vi "Reconnect.vi"(8 "error in (no error)":errorcluster, 11 "navX - I2C in":refnum<class "navX - I2C.lvclass">) -> (0 "error out":errorcluster, 3 "navX - I2C out":refnum<class "navX - I2C.lvclass">)   [LabVIEW 2015, in "navX Library v3.lvlib" / "navX - I2C.lvclass"]
uses:
  navX - I2C.lvclass
  navX - I2C.lvclass/navX - I2C.ctl
  navX - SPI_I2C ProcessingLoop/navX - SPI_I2C ProcessingLoop.lvclass
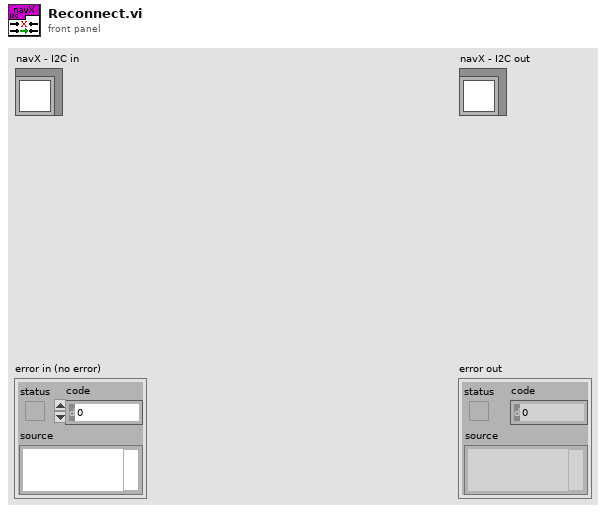
[diagram p1: front panel]
types:
  T1 = typedef "i2c_bus.ctl" = enum16{"I2C On-Board", "I2C MXP", "Invalid"}
  T2 = typedef "WPI_I2CDevRef.ctl" = cluster{"DevStatus":errorcluster, "Device Address":u8, "Handle":i32, "I2C Bus":T1}
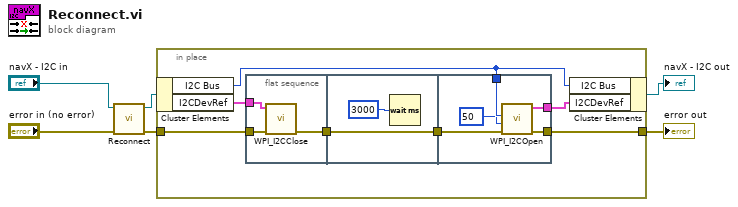
[diagram p0: block diagram]
diagram:
  n1 = call-parent "Reconnect.vi"("error in (no error)"="error in (no error)", "navX - Interface in"="navX - I2C in") -> ("error out"=w3:errorcluster, "navX - Interface out"=w4:refnum<class "navX - I2C.lvclass">)  [unwired: 8 in]
  n2 = in-place {
    in-place-border: [w13] -> w1
    in-place-border: w3 -> [w12]
    n3 = in-place-cluster #1(w4) -> ("I2C Bus"=w9:T1, "I2CDevRef"=w8:T2)
    n4 = flat-sequence {
      tunnel: w12 -> [w15]
      tunnel: w8 -> [w16]
      tunnel: [w14] -> w11
      tunnel: w11 -> [w18]
      tunnel: [w18] -> w10
      tunnel: [w23] -> w7
      tunnel: [w22] -> w13
      tunnel: w10 -> [w21]
      tunnel: w9 -> [w20]
      frame #0 {
        n5 = call <vilib>:"WPI_I2CClose.vi"("error in (no error)"=w15, "I2CDevRef"=w16) -> ("error out"=w14:errorcluster)  [unwired: 9 in]
      }
      frame #1 {
        n6 = Wait (ms)(milliseconds to wait=u32 3000) -> ()  [unwired: 1 out]
      }
      frame #2 {
        n7 = call <vilib>:"WPI_I2COpen.vi"("error in"=w21, "Device Address"=u8 50, "I2C Bus"=w20) -> ("error out"=w22:errorcluster, "I2CDevRef"=w23:T2)  [unwired: 7 in]
      }
    }
    n8 = in-place-cluster #1("I2C Bus"=w9, "I2CDevRef"=w7) -> (→"navX - I2C out":refnum<class "navX - I2C.lvclass">)
  }
  "error out" <- w1
